vi "Write byte order.vi"(8 "error in (no error)":errorcluster, 10 "byte order":dbl, 11 "DSFTransfer in":refnum<class "DSFTransfer.lvclass">) -> (0 "error out":errorcluster, 3 "DSFTransfer out":refnum<class "DSFTransfer.lvclass">)   [LabVIEW 2017, in "DSFTransfer.lvclass"]
uses:
  DSFTransfer.lvclass
  DSFTransfer.lvclass/DSFTransfer.ctl
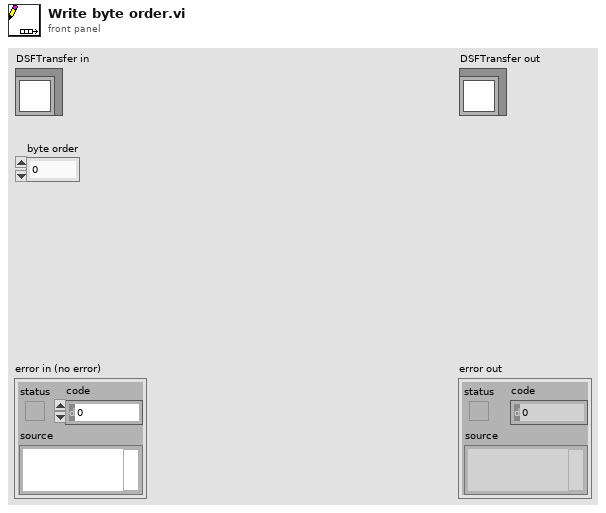
[diagram p1: front panel]
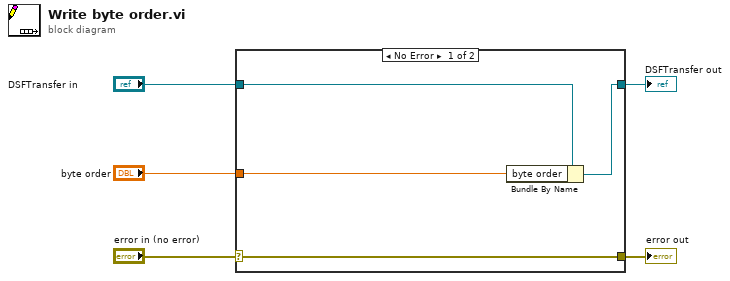
[diagram p0: block diagram]
diagram:
  n1 = case shown="No Error" "error in (no error)" {
    selector: "error in (no error)" -> [w9 w10]
    tunnel: [w9 w10] -> w4
    tunnel: [w7 w11] -> w2
    tunnel: "DSFTransfer in" -> [w8 w11]
    tunnel: "byte order" -> [w6 _]
    frame No Error {
      n2 = Bundle By Name(cluster=w8, "byte order"=w6) -> (w7:refnum<class "DSFTransfer.lvclass">)
    }
    frame Error {
    }
  }
  "error out" <- w4
  "DSFTransfer out" <- w2
